vi "Add_filename_suffix.vi"(0 "Filename":string, 1 "Suffix to add":string) -> (2 "Original Suffix":string, 3 "Filename out":string, 4 "Base name":string, 5 "Extension length":i32)   [LabVIEW 2011]
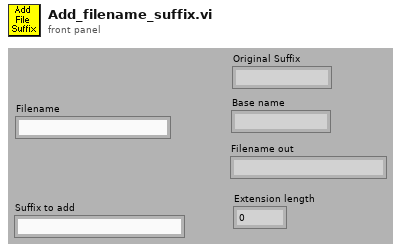
[diagram p1: front panel]
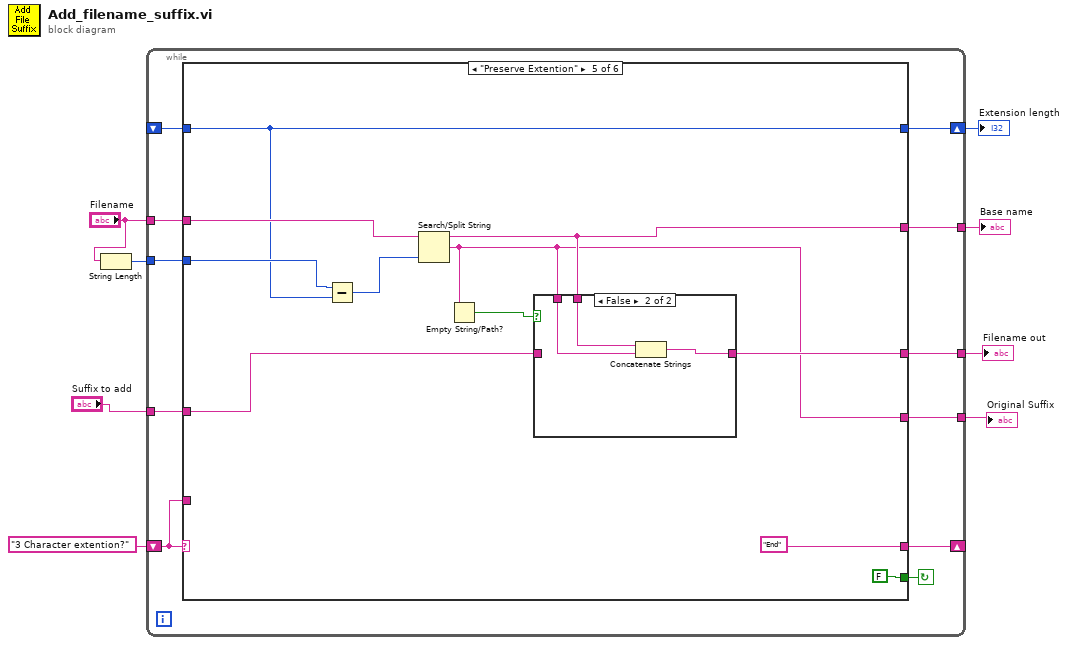
[diagram p0: block diagram]
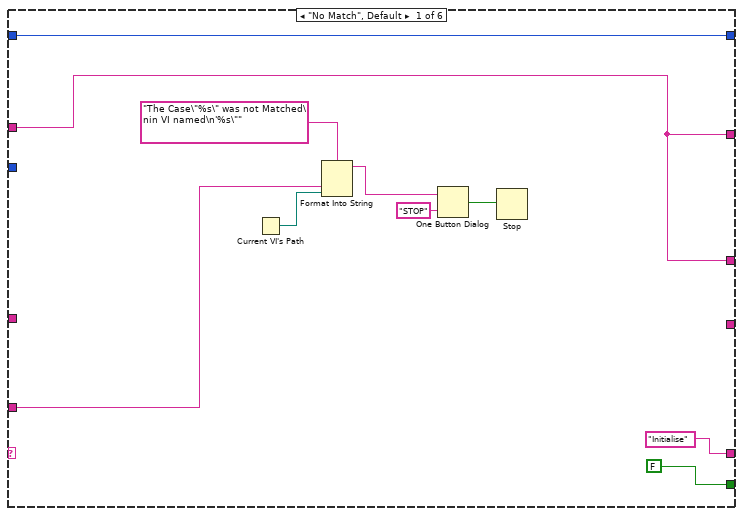
[diagram p2: hidden frame]
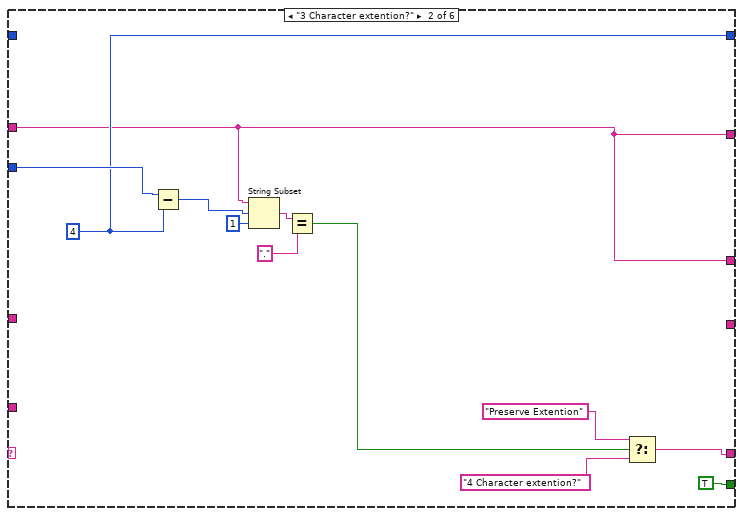
[diagram p3: hidden frame]
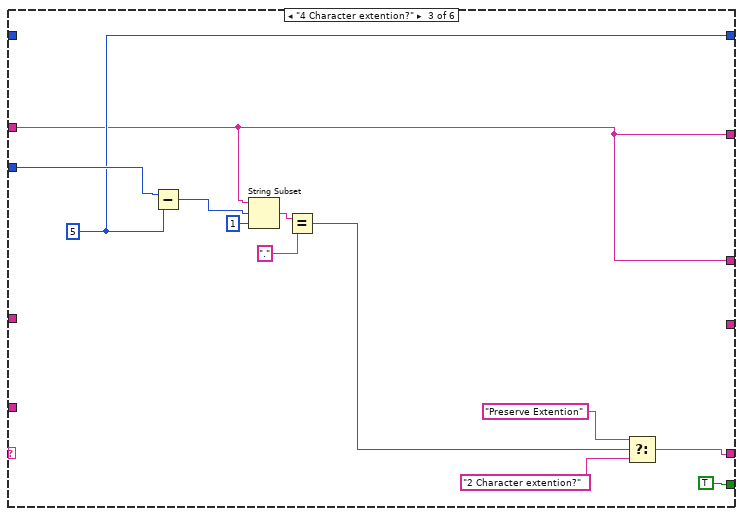
[diagram p4: hidden frame]
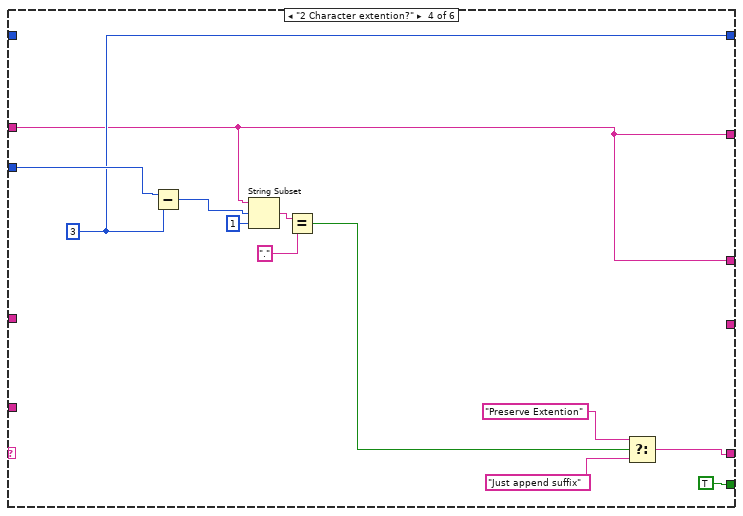
[diagram p5: hidden frame]
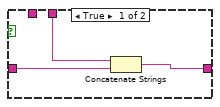
[diagram p6: hidden frame]
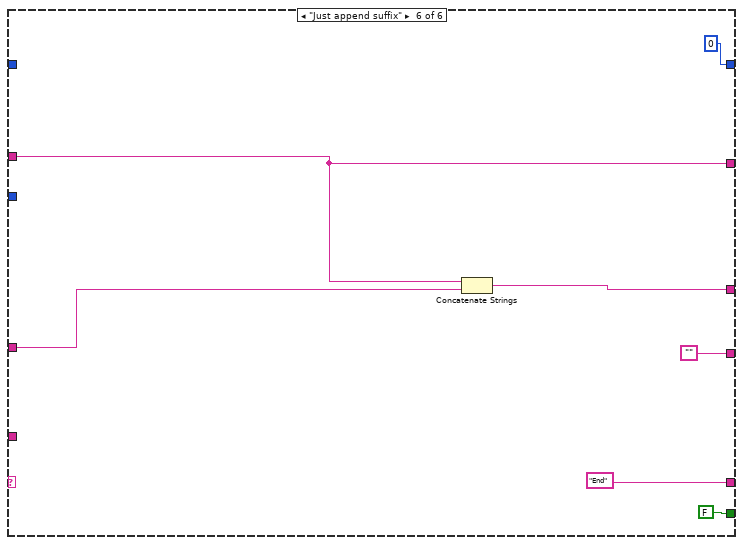
[diagram p7: hidden frame]
diagram:
  n1 = String Length(string="Filename") -> (length=w7:i32)
  n2 = while {
    shift-left: "3 Character extention?" -> [w17]
    shift-right: [w18] -> _
    tunnel: w7 -> [w16]
    tunnel: "Filename" -> [w15]
    tunnel: "Suffix to add" -> [w14]
    tunnel: [w13] -> w4
    shift-right: [w12] -> w3
    shift-left: _ -> [w11]
    tunnel: [w10] -> w2
    tunnel: [w9] -> w1
    stop <- w19 continue-if-true
    n3 = case shown="\"Preserve Extention\"" w17 {
      tunnel: [FALSE TRUE TRUE TRUE FALSE FALSE] -> w19
      tunnel: ["Initialise" w32 w44 w56 "End" "End"] -> w18
      tunnel: w17 -> [w24 _ _ _ _ _]
      tunnel: w16 -> [_ w40 w52 w64 w74 _]
      tunnel: w15 -> [w20 w30 w42 w54 w72 w84]
      tunnel: w14 -> [_ _ _ _ w68 w87]
      tunnel: [w20 w30 w42 w54 w71 w86] -> w13
      tunnel: [w21 w35 w47 w59 w70 0 ("y")] -> w12
      tunnel: w11 -> [w21 _ _ _ w70 _]
      tunnel: [w20 w30 w42 w54 w69 w84] -> w10
      tunnel: [_ _ _ _ w66 ""] -> w9
      frame "No Match", Default {
        n4 = Current VI's Path() -> (path=w23:path)
        n5 = Format Into String(format string="The Case\"%s\" was not Matched\nin VI named\n'%s\"" ("Format String"), w24, w23) -> (resulting string=w27:string)  [unwired: 2 in, 1 out]
        n6 = One Button Dialog(message=w27, button name ("OK")="STOP") -> (true=w25:bool)
        n7 = Stop(stop? (T)=w25) -> ()
      }
      frame "3 Character extention?" {
        w35 = 4 ("y")
        n8 = Subtract(x=w40, y=w35) -> (x-y=w37:i32)
        n9 = String Subset(string=w30, offset (0)=w37, length (rest)=1 ("length (rest)")) -> (substring=w36:string)
        n10 = Equal?(x=w36, y=".") -> (x = y?=w34:bool)
        n11 = Select(t="Preserve Extention", s=w34, f="4 Character extention?") -> (s? t:f=w32:string)
      }
      frame "4 Character extention?" {
        w47 = 5 ("y")
        n12 = Subtract(x=w52, y=w47) -> (x-y=w49:i32)
        n13 = String Subset(string=w42, offset (0)=w49, length (rest)=1 ("length (rest)")) -> (substring=w48:string)
        n14 = Equal?(x=w48, y=".") -> (x = y?=w46:bool)
        n15 = Select(t="Preserve Extention", s=w46, f="2 Character extention?") -> (s? t:f=w44:string)
      }
      frame "2 Character extention?" {
        w59 = 3 ("y")
        n16 = Subtract(x=w64, y=w59) -> (x-y=w61:i32)
        n17 = String Subset(string=w54, offset (0)=w61, length (rest)=1 ("length (rest)")) -> (substring=w60:string)
        n18 = Equal?(x=w60, y=".") -> (x = y?=w58:bool)
        n19 = Select(t="Preserve Extention", s=w58, f="Just append suffix") -> (s? t:f=w56:string)
      }
      frame "Preserve Extention" {
        n20 = Subtract(x=w74, y=w70) -> (x-y=w73:i32)
        n21 = Search/Split String(string=w72, offset (0)=w73) -> (substring before match=w69:string, match + rest of string=w66:string)  [unwired: 2 out]
        n22 = Empty String/Path?(string/path=w66) -> (empty?=w67:bool)
        n23 = case shown="False" w67 {
          tunnel: w66 -> [_ w82]
          tunnel: [w79 w81] -> w71
          tunnel: w69 -> [w78 w80]
          tunnel: w68 -> [w77 _]
          frame True {
            n24 = Concatenate Strings(w78, w77) -> (w79:string)
          }
          frame False {
            n25 = Concatenate Strings(w80, w82) -> (w81:string)
          }
        }
      }
      frame "Just append suffix" {
        n26 = Concatenate Strings(w84, w87) -> (w86:string)
      }
    }
  }
  "Filename out" <- w4
  "Extension length" <- w3
  "Base name" <- w2
  "Original Suffix" <- w1
